vi "SerialSendHLcmd.vi"(0 "Command":string, 1 "Axis configuration":u16(ring) items=["No axis", "X", "Y", "Z", "XY", "XYZ"], 5 "X in":dbl format="%#.4f", 7 "Y in":dbl format="%#.4f", 9 "Z in":dbl format="%#.4f", 11 "error in (no error)":errorcluster, 12 "Command type":enum16{"Query", "Where", "Imperative", "DU Y"}(ring)) -> (4 "Raw receive buffer":string, 6 "X out":dbl, 8 "Y out":dbl, 10 "Z out":dbl, 15 "error out":errorcluster)   [LabVIEW 2010]
uses:
  SerialGlobals.vi
  <vilib>/Instr/_visa.llb/VISA Configure Serial Port (Instr).vi
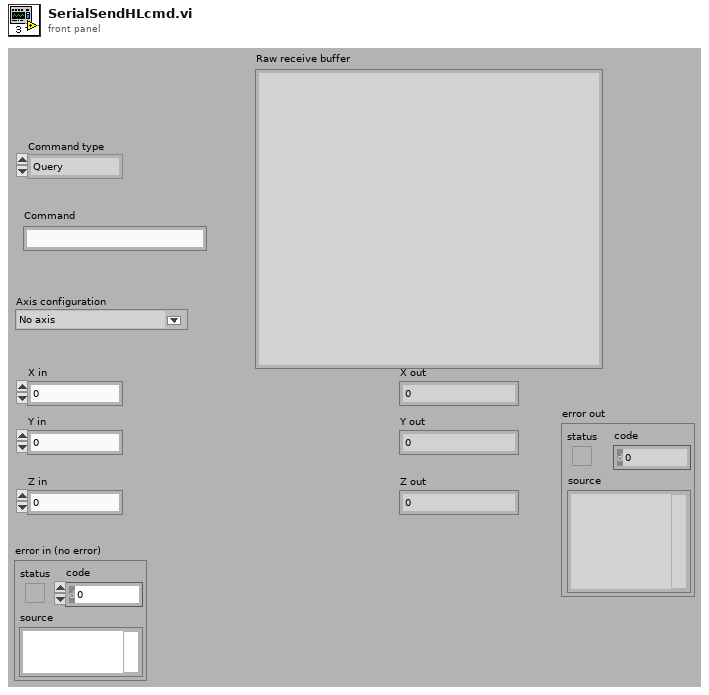
[diagram p1: front panel]
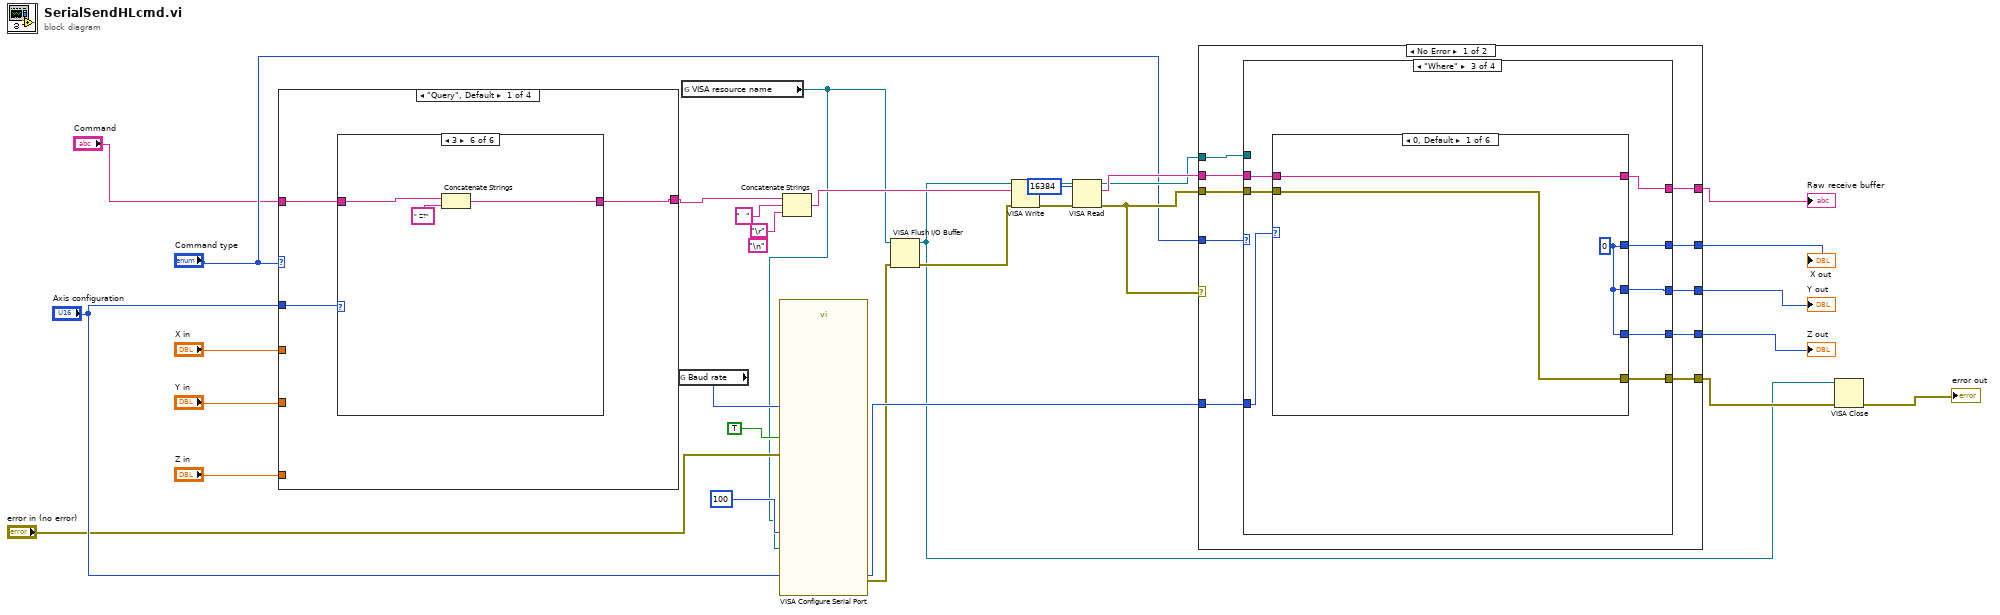
[diagram p0: block diagram]
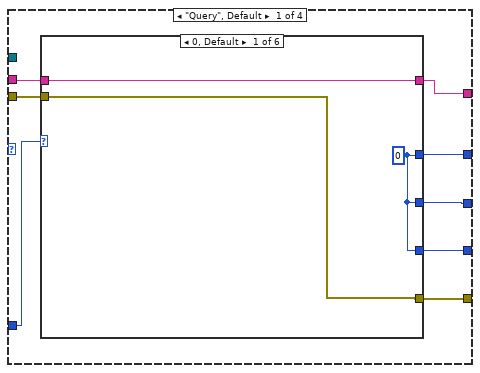
[diagram p2: hidden frame]
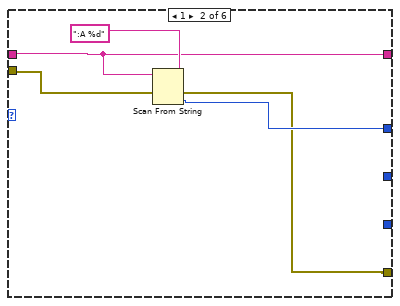
[diagram p3: hidden frame]
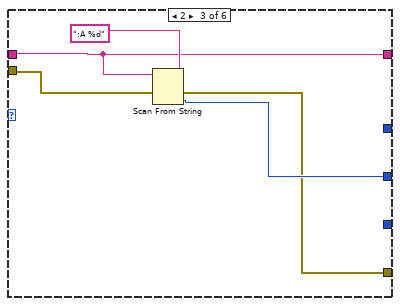
[diagram p4: hidden frame]
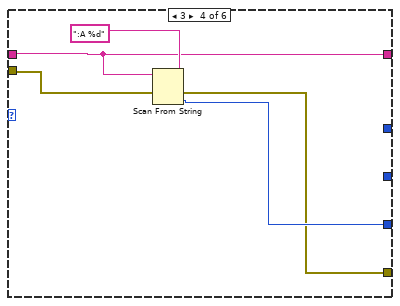
[diagram p5: hidden frame]
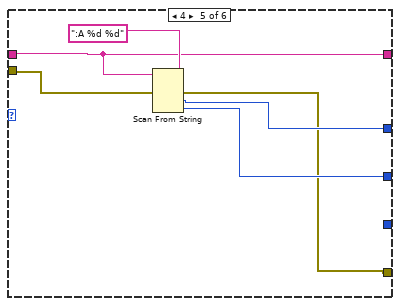
[diagram p6: hidden frame]
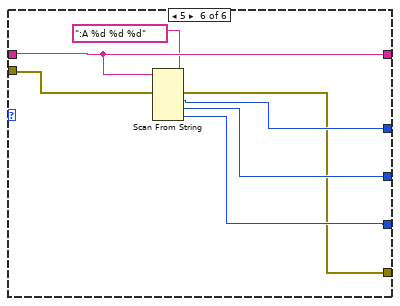
[diagram p7: hidden frame]
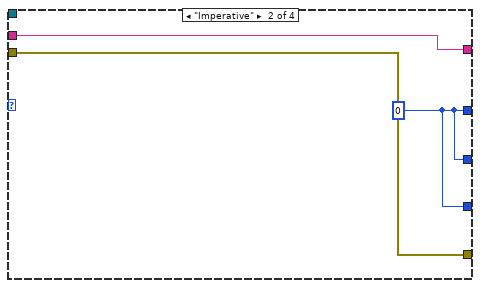
[diagram p8: hidden frame]
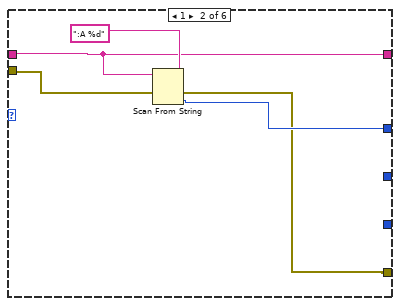
[diagram p9: hidden frame]
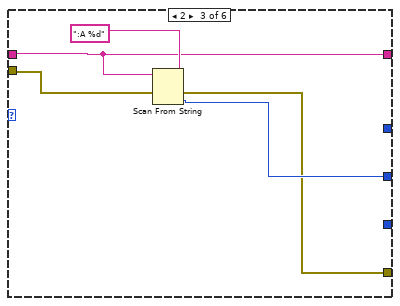
[diagram p10: hidden frame]
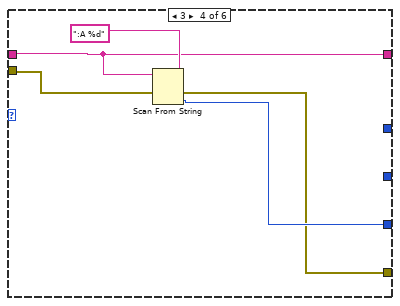
[diagram p11: hidden frame]
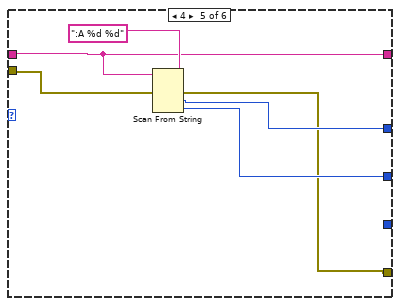
[diagram p12: hidden frame]
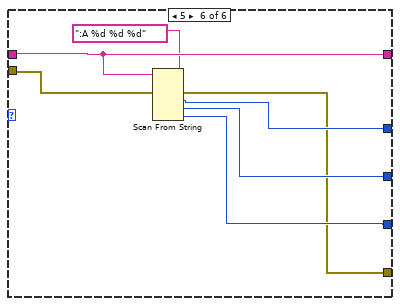
[diagram p13: hidden frame]
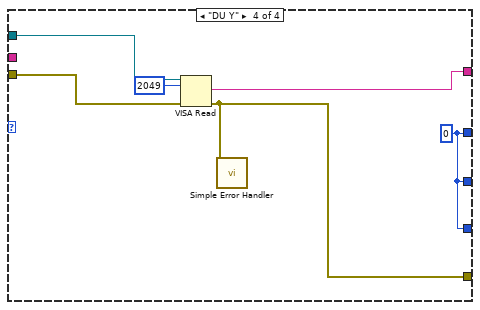
[diagram p14: hidden frame]
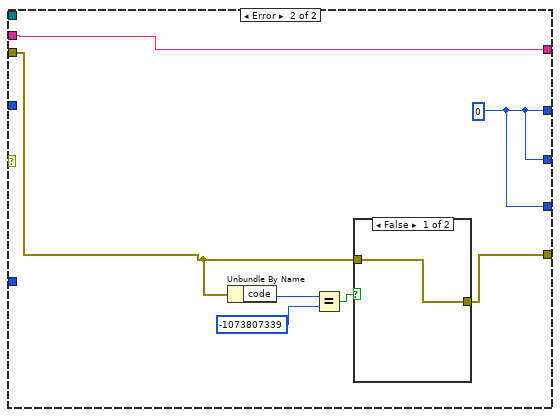
[diagram p15: hidden frame]
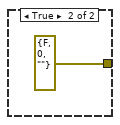
[diagram p16: hidden frame]
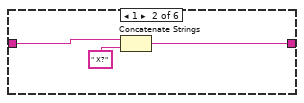
[diagram p18: hidden frame]
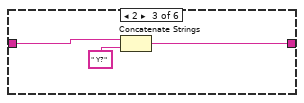
[diagram p19: hidden frame]
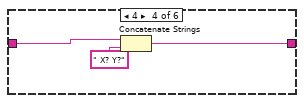
[diagram p20: hidden frame]
diagram:
  (unwired) "\n"
  n1 = case shown="\"Query\", Default" "Command type" {
    tunnel: "Command" -> [w32 w51 w74 _]
    tunnel: "Axis configuration" -> [w33 w52 w69 _]
    tunnel: "X in" -> [_ _ w73 _]
    tunnel: "Y in" -> [_ _ w72 _]
    tunnel: "Z in" -> [_ _ w71 _]
    tunnel: [w31 w50 w70 "DU Y "] -> w27
    frame "Query", Default {
      n2 = case shown="3" w33 {
        tunnel: w32 -> [w34 w37 w40 w43 w46 w49]
        tunnel: [w34 w35 w38 w41 w44 w47] -> w31
        frame 0, Default {
        }
        frame 1 {
          n3 = Concatenate Strings "Concatenate Strings"(w37, " X?") -> (w35:string)
        }
        frame 2 {
          n4 = Concatenate Strings "Concatenate Strings"(w40, " Y?") -> (w38:string)
        }
        frame 4 {
          n5 = Concatenate Strings "Concatenate Strings"(w43, " X? Y?") -> (w41:string)
        }
        frame 5 {
          n6 = Concatenate Strings "Concatenate Strings"(w46, " X? Y? Z?") -> (w44:string)
        }
        frame 3 {
          n7 = Concatenate Strings "Concatenate Strings"(w49, " Z?") -> (w47:string)
        }
      }
    }
    frame "Where" {
      n8 = case shown="5" w52 {
        tunnel: w51 -> [w53 w56 w59 w62 w65 w68]
        tunnel: [w53 w54 w57 w60 w63 w66] -> w50
        frame 0, Default {
        }
        frame 1 {
          n9 = Concatenate Strings "Concatenate Strings"(w56, " X ") -> (w54:string)
        }
        frame 2 {
          n10 = Concatenate Strings "Concatenate Strings"(w59, " Y ") -> (w57:string)
        }
        frame 4 {
          n11 = Concatenate Strings "Concatenate Strings"(w62, " X Y") -> (w60:string)
        }
        frame 5 {
          n12 = Concatenate Strings "Concatenate Strings"(w65, " X Y Z ") -> (w63:string)
        }
        frame 3 {
          n13 = Concatenate Strings "Concatenate Strings"(w68, " Z") -> (w66:string)
        }
      }
    }
    frame "Imperative" {
      n14 = case shown="5" w69 {
        tunnel: w74 -> [w75 w79 w83 w87 w92 w98]
        tunnel: w73 -> [_ w77 _ _ w89 w95]
        tunnel: w72 -> [_ _ w80 _ w88 w94]
        tunnel: w71 -> [_ _ _ w84 _ w93]
        tunnel: [w75 w76 w81 w85 w90 w96] -> w70
        frame 0, Default {
        }
        frame 1 {
          n15 = Format Into String "Format Into String"(format string="  X=%7.4f", initial string=w79, w77) -> (resulting string=w76:string)  [unwired: 1 in, 1 out]
        }
        frame 2 {
          n16 = Format Into String "Format Into String"(format string="  Y=%7.4f", initial string=w83, w80) -> (resulting string=w81:string)  [unwired: 1 in, 1 out]
        }
        frame 3 {
          n17 = Format Into String "Format Into String"(format string=" Z=%7.4f", initial string=w87, w84) -> (resulting string=w85:string)  [unwired: 1 in, 1 out]
        }
        frame 4 {
          n18 = Format Into String "Format Into String"(format string=" X=%7.4f  Y=%7.4f", initial string=w92, w89, w88) -> (resulting string=w90:string)  [unwired: 1 in, 1 out]
        }
        frame 5 {
          n19 = Format Into String "Format Into String"(format string=" X=%7.4f  Y=%7.4f Z=%7.4f", initial string=w98, w95, w94, w93) -> (resulting string=w96:string)  [unwired: 1 in, 1 out]
        }
      }
    }
    frame "DU Y" {
    }
  }
  n20 = global read "SerialGlobals.vi" "Baud rate"() -> (w2:u32)
  n21 = global read "SerialGlobals.vi" "VISA resource name"() -> (w1:refnum<visa-resource-name>)
  n22 = call-poly "VISA Configure Serial Port"("VISA resource name"=w1, "timeout (10sec)"=u32 100, "Enable Termination\nChar (T)"=TRUE ("Enable Termination\nChar (T)"), "baud rate (9600)"=w2, "error in (no error)"="error in (no error)") -> ("error out"=w9:errorcluster)  [unwired: 3 in, 7 out]
  n23 = Concatenate Strings "Concatenate Strings"(w27, "  ", "\r") -> (w24:string)
  n24 = VISA Flush I/O Buffer(VISA resource name=w1, error in (no error)=w9) -> (VISA resource name out=w5:refnum<visa-resource-name>, error out=w23:errorcluster)  [unwired: 1 out]
  n25 = VISA Write(VISA resource name=w5, write buffer=w24, error in (no error)=w23) -> (VISA resource name out=w22:refnum<visa-resource-name>, error out=w21:errorcluster)  [unwired: 1 out]
  n26 = VISA Read(VISA resource name=w22, byte count=u32 16384, error in (no error)=w21) -> (VISA resource name out=w12:refnum<visa-resource-name>, read buffer=w20:string, error out=w13:errorcluster)  [unwired: 1 out]
  n27 = case shown="No Error" w13 {
    tunnel: w20 -> [w109 w202]
    tunnel: "Command type" -> [w108 _]
    tunnel: "Axis configuration" -> [w107 _]
    tunnel: [w106 w202] -> w18
    tunnel: [w105 w203] -> w17
    tunnel: [w104 w203] -> w16
    tunnel: [w103 w203] -> w15
    tunnel: w13 -> [w102 w197]
    tunnel: [w101 w199] -> w10
    tunnel: w12 -> [w100 _]
    frame No Error {
      n28 = case shown="\"Where\"" w108 {
        tunnel: w109 -> [w116 w151 w158 _]
        tunnel: w107 -> [w117 _ w159 _]
        tunnel: [w115 w151 w157 w194] -> w106
        tunnel: [w113 w150 w155 w193] -> w105
        tunnel: [w112 w150 w154 w193] -> w104
        tunnel: [w111 w150 w153 w193] -> w103
        tunnel: w102 -> [w114 w149 w156 w195]
        tunnel: [w110 w149 w152 w191] -> w101
        tunnel: w100 -> [_ _ _ w196]
        frame "Query", Default {
          n29 = case shown="0, Default" w117 {
            tunnel: w116 -> [w120 w124 w129 w134 w140 w148]
            tunnel: [w120 w124 w129 w134 w140 w148] -> w115
            tunnel: w114 -> [w118 w123 w128 w133 w139 w147]
            tunnel: [w119 w122 _ _ w138 w146] -> w113
            tunnel: [w119 _ w127 _ w137 w145] -> w112
            tunnel: [w119 _ _ w132 _ w143] -> w111
            tunnel: [w118 w121 w126 w131 w136 w142] -> w110
            frame 0, Default {
              w119 = 0
            }
            frame 1 {
              n30 = Scan From String "Scan From String"(format string=":A %d", input string=w124, error in=w123) -> (error out=w121:errorcluster, output 1=w122:i32)  [unwired: 2 in, 2 out]
            }
            frame 2 {
              n31 = Scan From String "Scan From String"(format string=":A %d", input string=w129, error in=w128) -> (error out=w126:errorcluster, output 1=w127:i32)  [unwired: 2 in, 2 out]
            }
            frame 3 {
              n32 = Scan From String "Scan From String"(format string=":A %d", input string=w134, error in=w133) -> (error out=w131:errorcluster, output 1=w132:i32)  [unwired: 2 in, 2 out]
            }
            frame 4 {
              n33 = Scan From String "Scan From String"(format string=":A %d %d", input string=w140, error in=w139) -> (error out=w136:errorcluster, output 1=w138:i32, output 2=w137:i32)  [unwired: 3 in, 2 out]
            }
            frame 5 {
              n34 = Scan From String "Scan From String"(format string=":A %d %d %d", input string=w148, error in=w147) -> (error out=w142:errorcluster, output 1=w146:i32, output 2=w145:i32, output 3=w143:i32)  [unwired: 4 in, 2 out]
            }
          }
        }
        frame "Imperative" {
          w150 = 0
        }
        frame "Where" {
          n35 = case shown="0, Default" w159 {
            tunnel: w158 -> [w162 w166 w171 w176 w182 w190]
            tunnel: [w162 w166 w171 w176 w182 w190] -> w157
            tunnel: w156 -> [w160 w165 w170 w175 w181 w189]
            tunnel: [w161 w164 _ _ w180 w188] -> w155
            tunnel: [w161 _ w169 _ w179 w187] -> w154
            tunnel: [w161 _ _ w174 _ w185] -> w153
            tunnel: [w160 w163 w168 w173 w178 w184] -> w152
            frame 0, Default {
              w161 = 0
            }
            frame 1 {
              n36 = Scan From String "Scan From String"(format string=":A %d", input string=w166, error in=w165) -> (error out=w163:errorcluster, output 1=w164:i32)  [unwired: 2 in, 2 out]
            }
            frame 2 {
              n37 = Scan From String "Scan From String"(format string=":A %d", input string=w171, error in=w170) -> (error out=w168:errorcluster, output 1=w169:i32)  [unwired: 2 in, 2 out]
            }
            frame 3 {
              n38 = Scan From String "Scan From String"(format string=":A %d", input string=w176, error in=w175) -> (error out=w173:errorcluster, output 1=w174:i32)  [unwired: 2 in, 2 out]
            }
            frame 4 {
              n39 = Scan From String "Scan From String"(format string=":A %d %d", input string=w182, error in=w181) -> (error out=w178:errorcluster, output 1=w180:i32, output 2=w179:i32)  [unwired: 3 in, 2 out]
            }
            frame 5 {
              n40 = Scan From String "Scan From String"(format string=":A %d %d %d", input string=w190, error in=w189) -> (error out=w184:errorcluster, output 1=w188:i32, output 2=w187:i32, output 3=w185:i32)  [unwired: 4 in, 2 out]
            }
          }
        }
        frame "DU Y" {
          w193 = 0
          n41 = VISA Read(VISA resource name=w196, byte count=u32 2049, error in (no error)=w195) -> (read buffer=w194:string, error out=w191:errorcluster)  [unwired: 2 out]
          n42 = call <vilib>:"Simple Error Handler.vi"("error in (no error)"=w191) -> ()  [unwired: 1 in, 8 out]
        }
      }
    }
    frame Error {
      w203 = 0
      n43 = Unbundle By Name(w197) -> ("code"=w201:i32)
      n44 = Equal?(x=w201, y=-1073807339) -> (x = y?=w198:bool)
      n45 = case shown="False" w198 {
        tunnel: [w204 errorcluster {"status"=FALSE, "code"=0, "source"=""}] -> w199
        tunnel: w197 -> [w204 _]
        frame False {
        }
        frame True {
        }
      }
    }
  }
  "Raw receive buffer" <- w18
  "X out" <- w17
  "Y out" <- w16
  "Z out" <- w15
  n46 = VISA Close(VISA resource name=w5, error in (no error)=w10) -> (error out=→"error out":errorcluster)
